vi "Instr_InitObject.vi"(8 "error in (no error)":errorcluster, 9 "Instrument Configuration":variant, 10 "GPIB Address":string, 11 "LCRControl in":refnum<class "LCRControl.lvclass">) -> (0 "error out":errorcluster, 3 "LCRControl out":refnum<class "LCRControl.lvclass">)   [LabVIEW 2013, in "LCRControl.lvclass"]
uses:
  LCRControl.lvclass
  InstrControl.lvclass
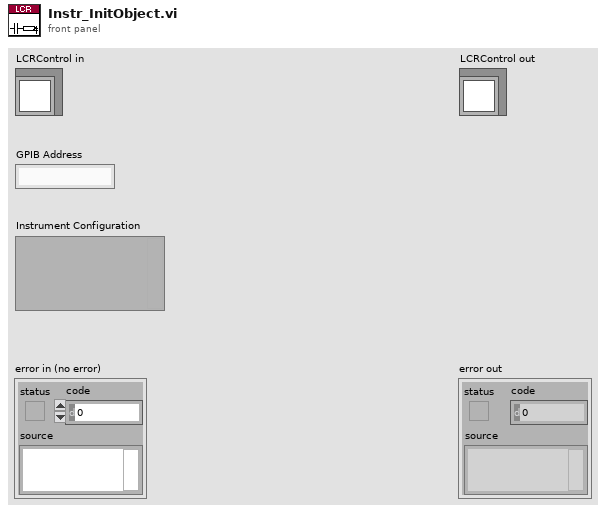
[diagram p1: front panel]
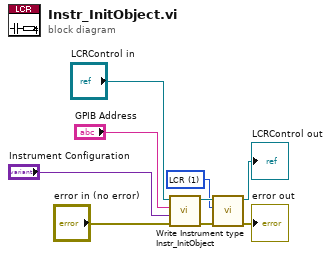
[diagram p0: block diagram]
diagram:
  w5 = u16 1 items=["Supply", "LCR"] ("Instrument type")
  n1 = call-parent "Instr_InitObject.vi"("error in (no error)"="error in (no error)", "Instrument Configuration"="Instrument Configuration", "GPIB Address"="GPIB Address", "InstrControl in"="LCRControl in") -> ("error out"=w4:errorcluster, "InstrControl out"=w7:refnum<class "LCRControl.lvclass">)  [unwired: 6 in]
  n2 = call-dynamic "Write Instrument type.vi"("error in (no error)"=w4, "Instrument type"=w5, "InstControl in"=w7) -> ("error out"=→"error out":errorcluster, "InstControl out"=→"LCRControl out":refnum<class "LCRControl.lvclass">)  [unwired: 7 in]
